vi "Graph_det_noise.vi"() -> ()   [LabVIEW 2015]
uses:
  <vilib>/Platform/TimedLoop/XDataNode/timing_clust.ctl
  <vilib>/Platform/TimedLoop/XDataNode/nitl_modes.ctl
  <vilib>/Platform/TimedLoop/XDataNode/wakeup.ctl
  <vilib>/rvi/Emulation/niFpgaGetClockAttributes.vi
  <vilib>/rvi/Emulation/niFpgaSctlEmulationGetInTimedLoop.vi
  <vilib>/rvi/Emulation/niFpgaEmulationReportErrorSimple.vi
  <vilib>/rvi/eio/common/nirviEmuTemplateMethod_errors.vi
  <vilib>/rvi/Emulation/niFpgaCriticalErrorInLSC.vi
  <vilib>/eio/EIONode/EIONode.xnode
  <vilib>/Platform/TimedLoop/XDataNode/XDataNode.xnode
  <vilib>/Platform/TimedLoop/XDataNode/XDNodeRunTimeDep.lvlib
panel:
  out "IO Module\\AI 3":u16
  out "IO Module\\AI 2":u16
  out "Tick Count(uSec)":u32
  out "IO Module\\AI 0":u16
  out "IO Module\\AI 1":u16
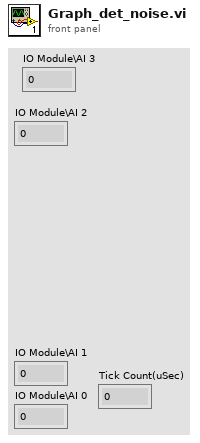
[diagram p1: front panel]
types:
  T1 = typedef "XDNodeRunTimeDep.lvlib/timing_clust.ctl" = cluster{"Expected End [f-1]":u64, "Actual End [f-1]":u64, "Finished Late? [f-1]":bool, "Expected End [i-1]":u64, "Actual End [i-1]":u64, "Finished Late? [i-1]":bool, "Expected Start [i]":u64, "Actual Start [i]":u64, "Expected Start [f]":u64, "Actual Start [f]":u64, "Source Name":string, "Structure Name":string, "Period":i64, "Deadline":i64, "Offset":i64, "Start":i64, "Priority":i32, "Timeout":i32, "Mode":T2, "Wakeup Reason":T3, "Error":errorcluster, "Source Type":string, "Secondary Source Type":string, "Global End Time":u64, "Global Start Time":u64, "Frame Duration":u64, "Iteration Duration":u64, "Assigned CPU":i32, "I/O Scan Engine Mode":u32}
  T2 = typedef "XDNodeRunTimeDep.lvlib/nitl_modes.ctl" = enum32{"No Change", "Process missed periods, maintain original phase", "Discard missed periods, maintain original phase", "Process missed periods, ignore original phase", "Discard missed periods, ignore original phase"}
  T3 = typedef "XDNodeRunTimeDep.lvlib/wakeup.ctl" = enum32{"Normal", "Aborted", "Asynchronous wakeup", "Timing source error", "Timed loop error", "Timeout"}
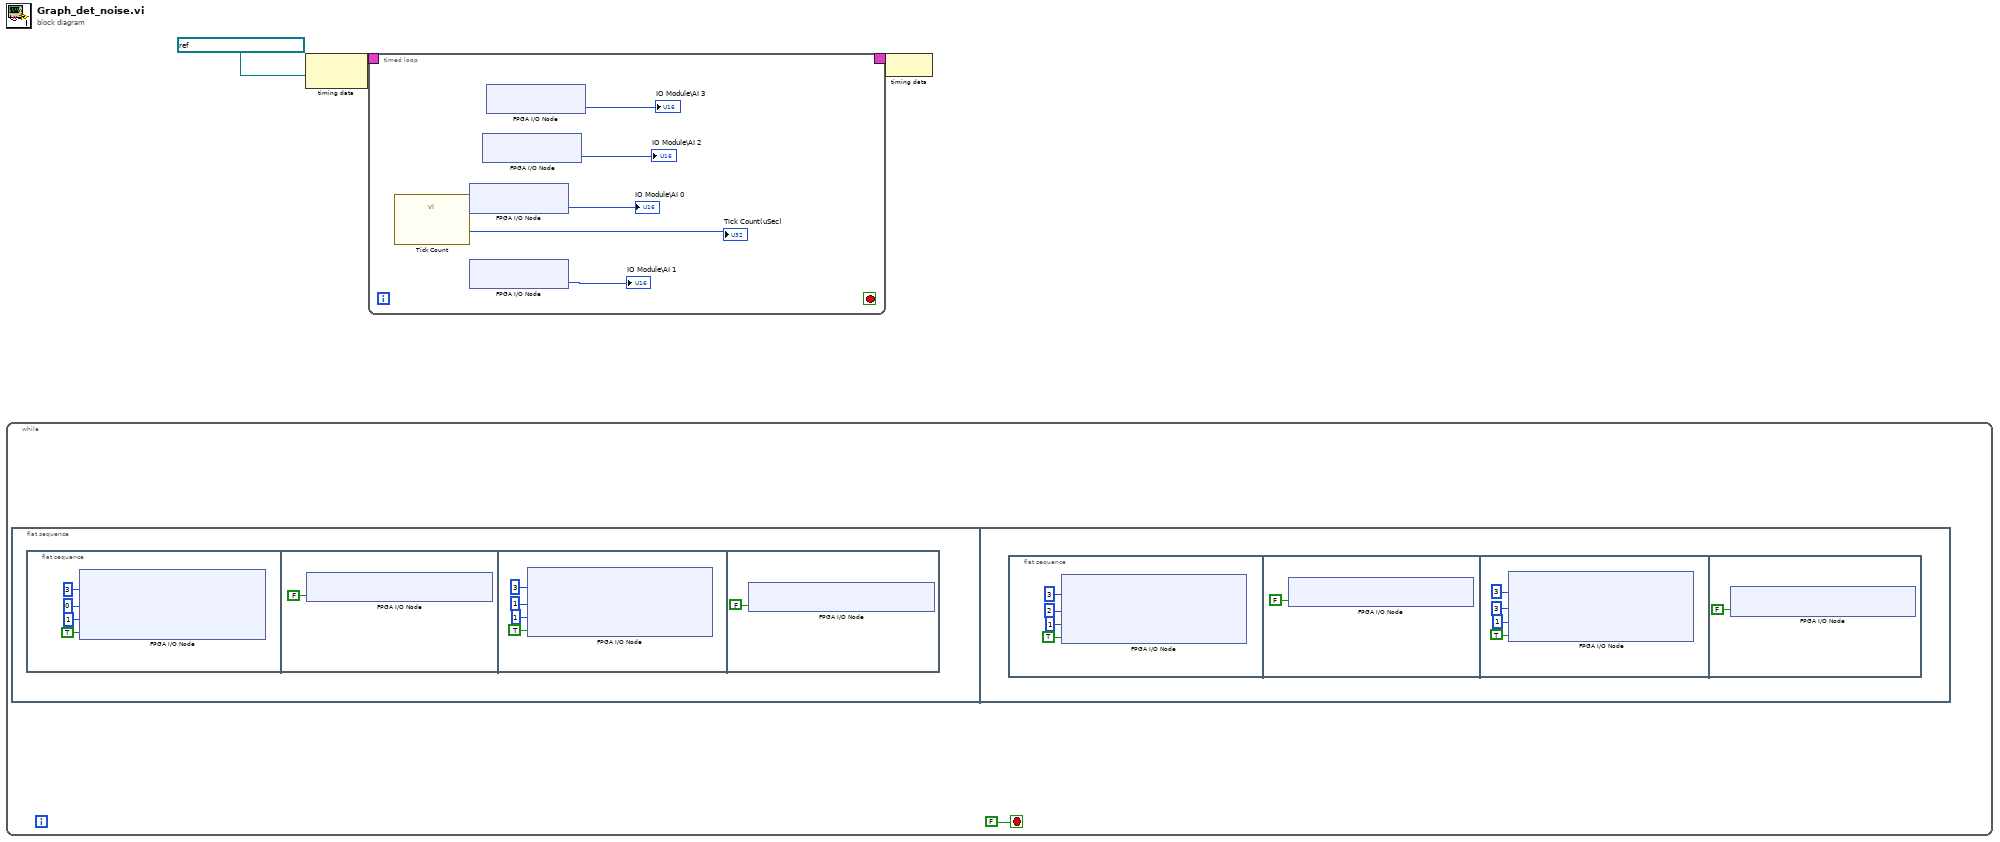
[diagram p0: block diagram]
diagram:
  n1 = while {
    stop <- FALSE stop-if-true
    n2 = flat-sequence {
      frame #0 {
        n3 = flat-sequence {
          frame #0 {
            n4 = xnode "FPGA I/O Node"("IO Module\\User Command"=u8 3 ("IO Module\\User Command"), "IO Module\\User Data 0"=u8 0 ("IO Module\\User Data 0"), "IO Module\\User Data 1"=u8 1 ("IO Module\\User Data 1"), "IO Module\\User Command Commit"=TRUE ("IO Module\\User Command Commit")) -> ()  [unwired: 4 in, 4 out]
          }
          frame #1 {
            n5 = xnode "FPGA I/O Node"("IO Module\\User Command Commit"=FALSE ("IO Module\\User Command Commit")) -> ()  [unwired: 1 in, 1 out]
          }
          frame #2 {
            n6 = xnode "FPGA I/O Node"("IO Module\\User Command"=u8 3 ("IO Module\\User Command"), "IO Module\\User Data 0"=u8 1 ("IO Module\\User Data 0"), "IO Module\\User Data 1"=u8 1 ("IO Module\\User Data 1"), "IO Module\\User Command Commit"=TRUE ("IO Module\\User Command Commit")) -> ()  [unwired: 4 in, 4 out]
          }
          frame #3 {
            n7 = xnode "FPGA I/O Node"("IO Module\\User Command Commit"=FALSE ("IO Module\\User Command Commit")) -> ()  [unwired: 1 in, 1 out]
          }
        }
      }
      frame #1 {
        n8 = flat-sequence {
          frame #0 {
            n9 = xnode "FPGA I/O Node"("IO Module\\User Command"=u8 3 ("IO Module\\User Command"), "IO Module\\User Data 0"=u8 2 ("IO Module\\User Data 0"), "IO Module\\User Data 1"=u8 1 ("IO Module\\User Data 1"), "IO Module\\User Command Commit"=TRUE ("IO Module\\User Command Commit")) -> ()  [unwired: 4 in, 4 out]
          }
          frame #1 {
            n10 = xnode "FPGA I/O Node"("IO Module\\User Command Commit"=FALSE ("IO Module\\User Command Commit")) -> ()  [unwired: 1 in, 1 out]
          }
          frame #2 {
            n11 = xnode "FPGA I/O Node"("IO Module\\User Command"=u8 3 ("IO Module\\User Command"), "IO Module\\User Data 0"=u8 3 ("IO Module\\User Data 0"), "IO Module\\User Data 1"=u8 1 ("IO Module\\User Data 1"), "IO Module\\User Command Commit"=TRUE ("IO Module\\User Command Commit")) -> ()  [unwired: 4 in, 4 out]
          }
          frame #3 {
            n12 = xnode "FPGA I/O Node"("IO Module\\User Command Commit"=FALSE ("IO Module\\User Command Commit")) -> ()  [unwired: 1 in, 1 out]
          }
        }
      }
    }
  }
  n13 = node-c288(refnum<k21> "IO Module\\Sample Clock" ("Source Name")) -> (w3:T1)
  n14 = timed-loop {
    timing: w3 -> [_]
    timing-out: [_] -> w2
    stop <- _ stop-if-true
    n15 = call "Tick Count"() -> ("Tick Count(uSec)"=→"Tick Count(uSec)":u32)
    n16 = xnode "FPGA I/O Node"() -> ("IO Module\\AI 0"=→"IO Module\\AI 0":u16)  [unwired: 1 in, 1 out]
    n17 = xnode "FPGA I/O Node"() -> ("IO Module\\AI 1"=→"IO Module\\AI 1":u16)  [unwired: 1 in, 1 out]
    n18 = xnode "FPGA I/O Node"() -> ("IO Module\\AI 2"=→"IO Module\\AI 2":u16)  [unwired: 1 in, 1 out]
    n19 = xnode "FPGA I/O Node"() -> ("IO Module\\AI 3"=→"IO Module\\AI 3":u16)  [unwired: 1 in, 1 out]
  }
  n20 = node-c288(w2) -> ()
